vi "baogao2.vi"() -> ()   [LabVIEW 2017]
panel:
  out "x":i32
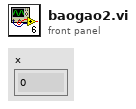
[diagram p1: front panel]
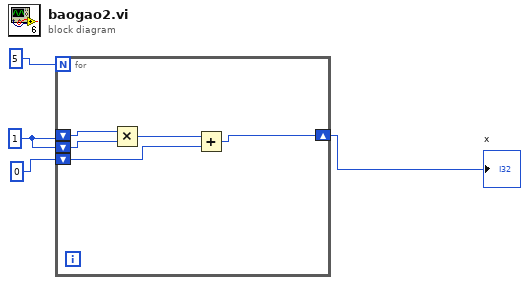
[diagram p0: block diagram]
diagram:
  w3 = 1
  n1 = for {
    N: 5 -> [_]
    shift-right: [w5] -> w2
    shift-left: w3 -> [w9]
    shift-left: w3 -> [w8]
    shift-left: 0 -> [w6]
    n2 = Multiply(x=w9, y=w8) -> (x*y=w7:i32)
    n3 = Add(x=w7, y=w6) -> (x+y=w5:i32)
  }
  "x" <- w2
